vi "fgm_all_in_one_loop.vi"() -> ()   [LabVIEW 2017]
uses:
  <vilib>/Platform/TimedLoop/XDataNode/timing_clust.ctl
  <vilib>/Platform/TimedLoop/XDataNode/nitl_modes.ctl
  <vilib>/Platform/TimedLoop/XDataNode/wakeup.ctl
  <vilib>/rvi/Emulation/niFpgaSctlEmulationGetInTimedLoop.vi
  <vilib>/rvi/Emulation/niFpgaEmulationReportErrorSimple.vi
  <vilib>/rvi/Emulation/niFpgaGetClockAttributes.vi
  <vilib>/rvi/Emulation/niFpgaCriticalErrorInLSC.vi
  <vilib>/Platform/TimedLoop/XDataNode/XDataNode.xnode
  <vilib>/Platform/TimedLoop/XDataNode/XDNodeRunTimeDep.lvlib
panel:
  in  "y0":fxp<+/-,32,3>[](array[numeric])=[0.0, 0.0, 0.0, 0.0, 0.0, 0.0, 0.0, 0.0, 0.0, 0.0, 0.0, 0.0]
  in  "z0,":fxp<+/-,32,3>[](array[numeric])=[0.0, 0.0, 0.0, 0.0, 0.0, 0.0, 0.0, 0.0, 0.0, 0.0, 0.0, 0.0]
  in  "y_i, x_k":fxp<+/-,32,3>[](array[numeric])=[0.0, 0.0, 0.0, 0.0, 0.0, 0.0, 0.0, 0.0, 0.0, 0.0, 0.0, 0.0]
  in  "SLMAX":fxp<+/-,18,5>
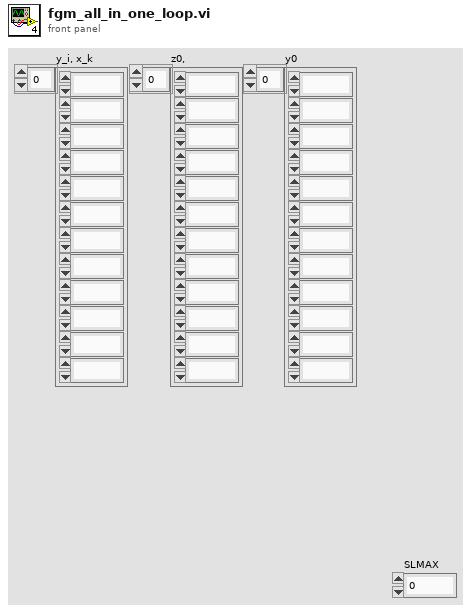
[diagram p1: front panel]
types:
  T1 = typedef "XDNodeRunTimeDep.lvlib/timing_clust.ctl" = cluster{"Expected End [f-1]":u64, "Actual End [f-1]":u64, "Finished Late? [f-1]":bool, "Expected End [i-1]":u64, "Actual End [i-1]":u64, "Finished Late? [i-1]":bool, "Expected Start [i]":u64, "Actual Start [i]":u64, "Expected Start [f]":u64, "Actual Start [f]":u64, "Source Name":string, "Structure Name":string, "Period":i64, "Deadline":i64, "Offset":i64, "Start":i64, "Priority":i32, "Timeout":i32, "Mode":T2, "Wakeup Reason":T3, "Error":errorcluster, "Source Type":string, "Secondary Source Type":string, "Global End Time":u64, "Global Start Time":u64, "Frame Duration":u64, "Iteration Duration":u64, "Assigned CPU":i32, "I/O Scan Engine Mode":u32}
  T2 = typedef "XDNodeRunTimeDep.lvlib/nitl_modes.ctl" = enum32{"No Change", "Process missed periods, maintain original phase", "Discard missed periods, maintain original phase", "Process missed periods, ignore original phase", "Discard missed periods, ignore original phase"}
  T3 = typedef "XDNodeRunTimeDep.lvlib/wakeup.ctl" = enum32{"Normal", "Aborted", "Asynchronous wakeup", "Timing source error", "Timed loop error", "Timeout"}
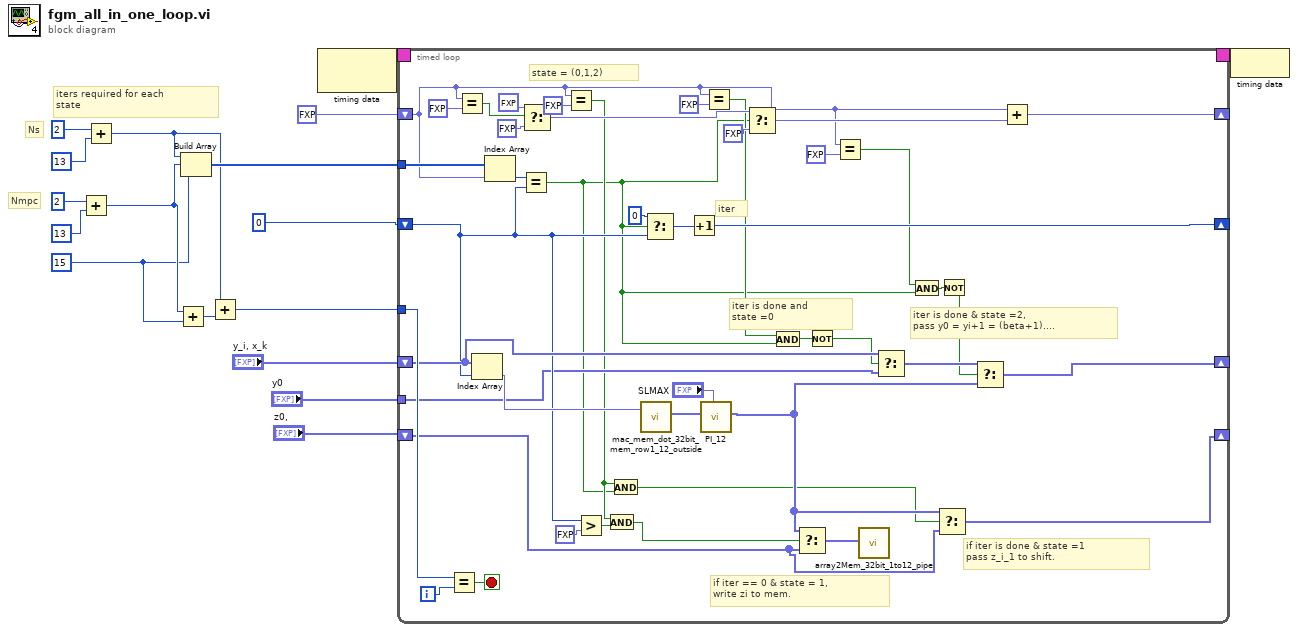
[diagram p0: block diagram]
diagram:
  w7 = i16 15
  # "iters required for each\nstate"
  # "Nmpc"
  # "Ns"
  n1 = Add(x=i16 2, y=i16 13) -> (x+y=w8:i16)
  n2 = Add(x=i16 2, y=i16 13) -> (x+y=w5:i16)
  n3 = Add(x=w8, y=w7) -> (x+y=w6:i16)
  n4 = Build Array(w5, w8, w7) -> (w9:i16[])
  n5 = Add(x=w5, y=w6) -> (x+y=w4:i16)
  n6 = node-c288() -> (w17:T1)  [unwired: 1 in]
  n7 = timed-loop {
    timing: w17 -> [_]
    timing-out: [_] -> w16
    shift-right: [w48] -> _
    shift-left: fxp<+/-,3,3> 0.0 -> [w22]
    shift-right: [w50] -> _
    shift-left: i16 0 -> [w33]
    tunnel: w9 -> [w57]
    tunnel: w4 -> [w51]
    shift-right: [w26] -> _
    shift-left: "y_i, x_k" -> [w41]
    shift-right: [w29] -> _
    shift-left: "z0," -> [w30]
    tunnel: "y0" -> [w31]
    i -> [w52]
    stop <- w53 stop-if-true
    # "if iter is done & state =1\npass z_i_1 to shift."
    # "iter is done & state =2,\npass y0 = yi+1 = (beta+1)...."
    # "if iter == 0 & state = 1,\nwrite zi to mem."
    # "iter is done and \nstate =0"
    # "iter"
    # "state = (0,1,2)"
    n8 = Equal?(x=w51, y=w52) -> (x = y?=w53:bool)
    n9 = Equal?(x=w22, y=fxp<+,2,2> 2.0) -> (x = y?=w54:bool)
    n10 = Index Array(array=w41, index=w33) -> (element=w42:fxp<+/-,32,3>)
    n11 = Index Array(array=w57, index=w22) -> (element=w56:i16)
    n12 = Equal?(x=w56, y=w33) -> (x = y?=w19:bool)
    n13 = Select(t=fxp<+/-,1,1> -1.0, s=w54, f=fxp<+,1,1> 1.0) -> (s? t:f=w46:fxp<+/-,2,2>)
    n14 = Equal?(x=w22, y=fxp<+,1,1> 1.0) -> (x = y?=w20:bool)
    n15 = Greater?(x=w33, y=fxp<+,2,2> 0.0) -> (0:w35:bool)
    n16 = And(x=w20, y=w35) -> (x .and. y?=w32:bool)
    n17 = And(x=w20, y=w19) -> (x .and. y?=w18:bool)
    n18 = call "mac_mem_dot_32bit_mem_row1_12_outside.vi"("x_i"=w42) -> ("appended array"=w44:fxp<+/-,32,3>[])  [unwired: 18 in]
    n19 = Select(t=i16 0, s=w19, f=w33) -> (s? t:f=w49:i16)
    n20 = Increment(x=w49) -> (x+1=w50:i16)
    n21 = call "PI_12.vi"("SLMAX"="SLMAX", "array in"=w44) -> ("appended array"=w28:fxp<+/-,32,3>[])  [unwired: 9 in]
    n22 = Equal?(x=w22, y=fxp<+,2,2> 0.0) -> (x = y?=w39:bool)
    n23 = Select(t=w46, s=w19, f=fxp<+,1,1> 0.0) -> (s? t:f=w59:fxp<+/-,2,2>)
    n24 = And(x=w39, y=w19) -> (x .and. y?=w38:bool)
    n25 = Select(t=w28, s=w32, f=w30) -> (s? t:f=w43:fxp<+/-,32,3>[])
    n26 = Not(x=w38) -> (.not. x?=w37:bool)
    n27 = Equal?(x=w22, y=fxp<+,2,2> 2.0) -> (x = y?=w21:bool)
    n28 = call "array2Mem_32bit_1to12_pipe.vi"("array in"=w43) -> ()  [unwired: 11 in]
    n29 = Select(t=w41, s=w37, f=w31) -> (s? t:f=w27:fxp<+/-,32,3>[])
    n30 = And(x=w21, y=w19) -> (x .and. y?=w25:bool)
    n31 = Select(t=w28, s=w18, f=w30) -> (s? t:f=w29:fxp<+/-,32,3>[])
    n32 = Not(x=w25) -> (.not. x?=w24:bool)
    n33 = Select(t=w27, s=w24, f=w28) -> (s? t:f=w26:fxp<+/-,32,3>[])
    n34 = Add(x=w22, y=w59) -> (x+y=w48:fxp<+/-,3,3>)
  }
  n35 = node-c288(w16) -> ()
